vi "Calculate Axis Value.vi"(9 "Plot Range":cluster{"Max":sgl, "Min":sgl}, 10 "Set Range":cluster{"Max":sgl, "Min":sgl}, 11 "Auto Range?":bool) -> (0 "Actual Range Out":cluster{"Max":sgl, "Min":sgl}, 2 "Translate Out":sgl, 3 "Scale Out":sgl)   [LabVIEW 2020, in "3D Plot.lvclass"]
uses:
  <vilib>/Math Plots/3D Math Plots/3D Plot/3D Plot/3D Plot.lvclass
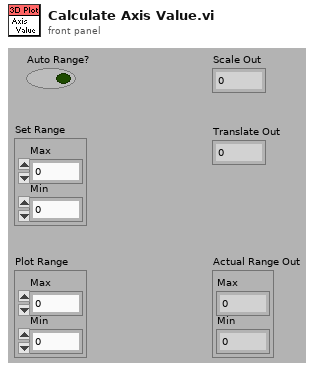
[diagram p1: front panel]
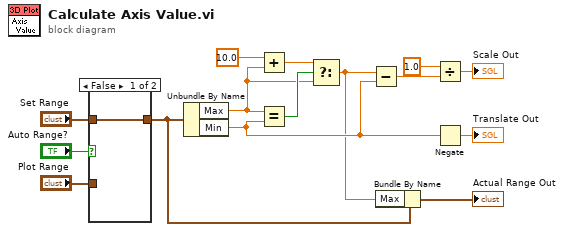
[diagram p0: block diagram]
diagram:
  n1 = case shown="False" "Auto Range?" {
    tunnel: [w16 w17] -> w3
    tunnel: "Plot Range" -> [_ w17]
    tunnel: "Set Range" -> [w16 _]
    frame False {
    }
    frame True {
    }
  }
  n2 = Unbundle By Name(w3) -> ("Max"=w4:sgl, "Min"=w5:sgl)
  n3 = Add(x=sgl 10.0 ("t"), y=w4) -> (x+y=w6:sgl)
  n4 = Equal?(x=w4, y=w5) -> (x = y?=w8:bool)
  n5 = Select(t=w6, s=w8, f=w4) -> (s? t:f=w1:sgl)
  n6 = Subtract(x=w1, y=w5) -> (x-y=w12:sgl)
  n7 = Bundle By Name(cluster=w3, "Max"=w1) -> (→"Actual Range Out":cluster{"Max":sgl, "Min":sgl})
  n8 = Divide(x=sgl 1.0 ("Numeric"), y=w12) -> (x/y=→"Scale Out":sgl)
  n9 = Negate(x=w5) -> (-x=→"Translate Out":sgl)
